vi "Cleanup Plot for Presentation-Paper.vi"(9 "Y Scale.Range:Minor Increment":dbl=0.5, 10 "X Scale.Range:Minor Increment":dbl=0.25, 11 "XY Graph Reference":refnum<vi>) -> (3 "reference out":refnum<vi>)   [LabVIEW 2010]
panel:
  in  "X Scale.Unit Label.Font:Size":u32=56
  in  "X Scale.Name Label.Font:Size":u32=60
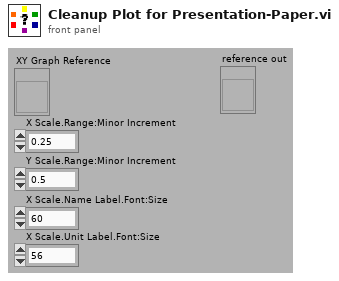
[diagram p1: front panel]
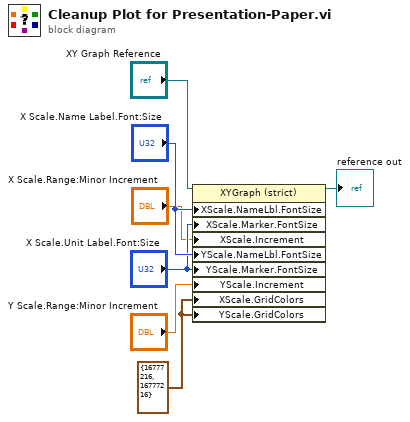
[diagram p0: block diagram]
diagram:
  w4 = cluster{"Color Box":u32, "Color Box 2":u32} {"Color Box"=16777216, "Color Box 2"=16777216}
  n1 = property on="Property Node" class="XYGraph (strict)"(reference="XY Graph Reference", "XScale.NameLbl.FontSize"="X Scale.Name Label.Font:Size", "XScale.Marker.FontSize"="X Scale.Unit Label.Font:Size", "XScale.Increment"="X Scale.Range:Minor Increment", "YScale.NameLbl.FontSize"="X Scale.Name Label.Font:Size", "YScale.Marker.FontSize"="X Scale.Unit Label.Font:Size", "YScale.Increment"="Y Scale.Range:Minor Increment", "XScale.GridColors"=w4, "YScale.GridColors"=w4) -> (reference out=→"reference out":refnum<vi>)  [unwired: 1 in, 1 out]
